vi "General CMD Operations.vi"(8 "error in (no error)":errorcluster, 10 "Message In":refnum<class "Message.lvclass">, 11 "System Actor in":refnum<class "System Actor.lvclass">) -> (0 "error out":errorcluster, 2 "Stop":bool, 3 "System Actor out":refnum<class "System Actor.lvclass">)   [LabVIEW 2024, in "System Actor.lvclass"]
uses:
  System Actor.lvclass
  Message/Message.lvclass
  Message/Message.lvclass/Message.ctl
  Message/Public Data/Read General CMD.vi
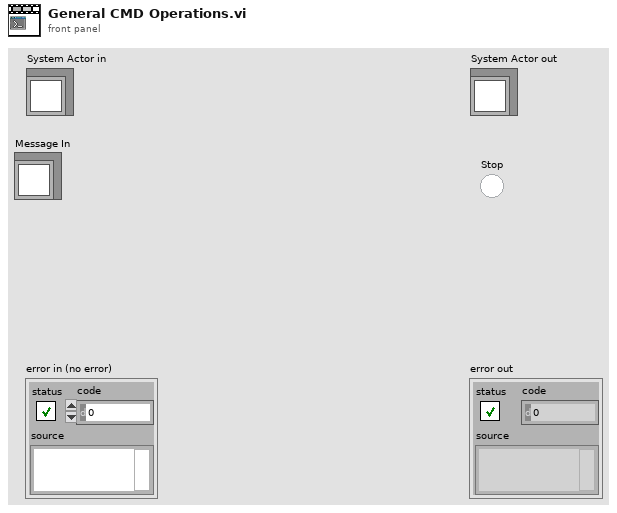
[diagram p1: front panel]
types:
  T1 = typedef "General CMD.ctl" = enum16{"None", "Stop", "Abort", "Running Task", "Running Batch Tasks", "Task Self Running", "Emergency Stop", "Subscribe", "UnSubscribe", "Pause", "Receive Parameters", "Active", "Resume"}
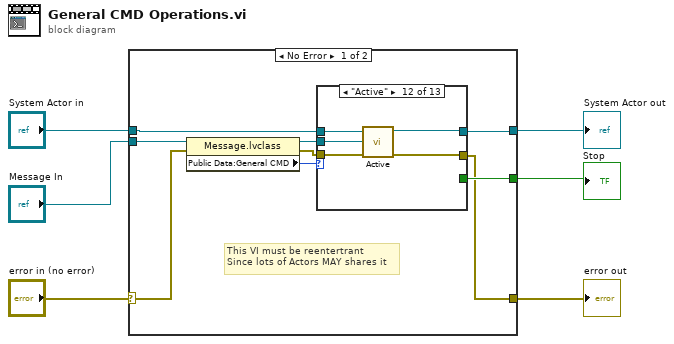
[diagram p0: block diagram]
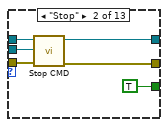
[diagram p3: hidden frame]
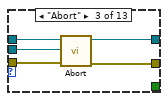
[diagram p4: hidden frame]
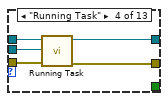
[diagram p5: hidden frame]
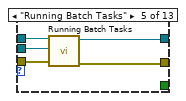
[diagram p6: hidden frame]
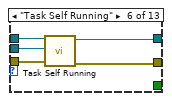
[diagram p7: hidden frame]
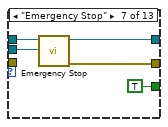
[diagram p8: hidden frame]
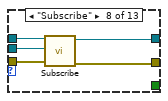
[diagram p9: hidden frame]
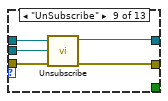
[diagram p10: hidden frame]
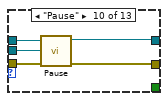
[diagram p11: hidden frame]
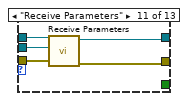
[diagram p12: hidden frame]
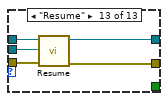
[diagram p13: hidden frame]
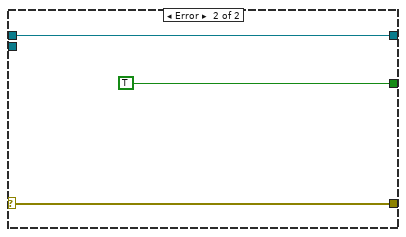
[diagram p14: hidden frame]
diagram:
  n1 = case shown="No Error" "error in (no error)" {
    selector: "error in (no error)" -> [w9 w81]
    tunnel: [w8 w81] -> w6
    tunnel: [w11 w80] -> w4
    tunnel: "System Actor in" -> [w12 w80]
    tunnel: [w10 TRUE] -> w1
    tunnel: "Message In" -> [w7 _]
    frame No Error {
      # "This VI must be reentertrant\nSince lots of Actors MAY shares it"
      n2 = property class="Message.lvclass"(reference=w7, error in=w9) -> (reference out=w14:refnum<class "Message.lvclass">, error out=w13:errorcluster, "Public Data:General CMD"=w15:T1)
      n3 = case shown="\"Active\"" w15 {
        tunnel: w12 -> [w17 w22 w28 w33 w38 w43 w47 w53 w58 w63 w68 w73 w78]
        tunnel: w14 -> [_ w21 w27 w31 w37 w39 w46 w51 w57 w62 w67 w71 w76]
        tunnel: w13 -> [w16 w18 w26 w30 w36 w41 _ w50 w56 w61 w66 w70 w75]
        tunnel: [w17 w20 w25 w32 w34 w42 w45 w52 w55 w59 w64 w72 w77] -> w11
        tunnel: [w16 w19 w24 w29 w35 w40 w44 w49 w54 w60 w65 w69 w74] -> w8
        tunnel: [_ TRUE _ _ _ _ TRUE _ _ _ _ _ _] -> w10
        frame "None", Default {
        }
        frame "Stop" {
          n4 = call-dynamic "Stop CMD.vi"("error in (no error)"=w18, "Message In"=w21, "System Actor in"=w22) -> ("error out"=w19:errorcluster, "System Actor out"=w20:refnum<class "System Actor.lvclass">)  [unwired: 7 in]
        }
        frame "Abort" {
          n5 = call-dynamic "Abort.vi"("error in (no error)"=w26, "Message In"=w27, "System Actor in"=w28) -> ("error out"=w24:errorcluster, "System Actor out"=w25:refnum<class "System Actor.lvclass">)  [unwired: 7 in]
        }
        frame "Running Task" {
          n6 = call-dynamic "Running Task.vi"("error in (no error)"=w30, "Message In"=w31, "System Actor in"=w33) -> ("error out"=w29:errorcluster, "System Actor out"=w32:refnum<class "System Actor.lvclass">)  [unwired: 7 in]
        }
        frame "Running Batch Tasks" {
          n7 = call-dynamic "Running Batch Tasks.vi"("error in (no error)"=w36, "Message In"=w37, "System Actor in"=w38) -> ("error out"=w35:errorcluster, "System Actor out"=w34:refnum<class "System Actor.lvclass">)  [unwired: 7 in]
        }
        frame "Task Self Running" {
          n8 = call-dynamic "Task Self Running.vi"("error in (no error)"=w41, "Message In"=w39, "System Actor in"=w43) -> ("error out"=w40:errorcluster, "System Actor out"=w42:refnum<class "System Actor.lvclass">)  [unwired: 7 in]
        }
        frame "Emergency Stop" {
          n9 = call-dynamic "Emergency Stop.vi"("Message In"=w46, "System Actor in"=w47) -> ("error out"=w44:errorcluster, "System Actor out"=w45:refnum<class "System Actor.lvclass">)  [unwired: 8 in]
        }
        frame "Subscribe" {
          n10 = call-dynamic "Subscribe.vi"("error in (no error)"=w50, "Message In"=w51, "System Actor in"=w53) -> ("error out"=w49:errorcluster, "System Actor out"=w52:refnum<class "System Actor.lvclass">)  [unwired: 7 in]
        }
        frame "UnSubscribe" {
          n11 = call-dynamic "Unsubscribe.vi"("error in (no error)"=w56, "Message In"=w57, "System Actor in"=w58) -> ("error out"=w54:errorcluster, "System Actor out"=w55:refnum<class "System Actor.lvclass">)  [unwired: 7 in]
        }
        frame "Pause" {
          n12 = call-dynamic "Pause.vi"("error in (no error)"=w61, "Message In"=w62, "System Actor in"=w63) -> ("error out"=w60:errorcluster, "System Actor out"=w59:refnum<class "System Actor.lvclass">)  [unwired: 7 in]
        }
        frame "Receive Parameters" {
          n13 = call-dynamic "Receive Parameters.vi"("error in (no error)"=w66, "Message In"=w67, "System Actor in"=w68) -> ("error out"=w65:errorcluster, "System Actor out"=w64:refnum<class "System Actor.lvclass">)  [unwired: 7 in]
        }
        frame "Active" {
          n14 = call-dynamic "Active.vi"("error in (no error)"=w70, "Message In"=w71, "System Actor in"=w73) -> ("error out"=w69:errorcluster, "System Actor out"=w72:refnum<class "System Actor.lvclass">)  [unwired: 7 in]
        }
        frame "Resume" {
          n15 = call-dynamic "Resume.vi"("error in (no error)"=w75, "Message In"=w76, "System Actor in"=w78) -> ("error out"=w74:errorcluster, "System Actor out"=w77:refnum<class "System Actor.lvclass">)  [unwired: 7 in]
        }
      }
    }
    frame Error {
    }
  }
  "error out" <- w6
  "System Actor out" <- w4
  "Stop" <- w1
